vi "Init(Config) String Control Sink.vi"(7 "Str Refnum":refnum<vi>, 8 "error in (no error)":errorcluster, 9 "iName":string, 10 "iType":string) -> (0 "error out":errorcluster, 3 "String Control Sink out":refnum<class "String Control Sink.lvclass">)   [LabVIEW 2016, in "Stream Log.lvlib" / "String Control Sink.lvclass"]
doc: "--\nCopyright © 2017 Composed SystemsI All rights reserved.\n\nAuthor: Jon McBee <jon.mcbee@composed.io>\n\nThis library is provided \"AS IS\" ,WITHOUT WARRANTIES OR\nCONDITIONS OF ANY KIND, either express or implied.\n\nComposed Systems -- composed.io\n\nStream 0.0.1.1\nJon McBee - Composed Systems\nCopyright (c) 2017, Composed Systems"
uses:
  <userlib>/Composed Systems/Stream/Log/String Control Sink/String Control Sink.lvclass
  C:/Program Files (x86)/National Instruments/LabVIEW 2016/user.lib/Composed Systems/Stream/Actor/Actor Class/Ancestral Actor.lvclass
  <userlib>/Composed Systems/Stream/Actor/Actor Class/Ancestral Actor.lvclass/Ancestral Actor.ctl
  <userlib>/Composed Systems/Stream/Log/String Control Sink/String Control Sink.lvclass/String Control Sink.ctl
  <userlib>/Composed Systems/Stream/Actor/Actor Class/Ancestral Actor.lvclass
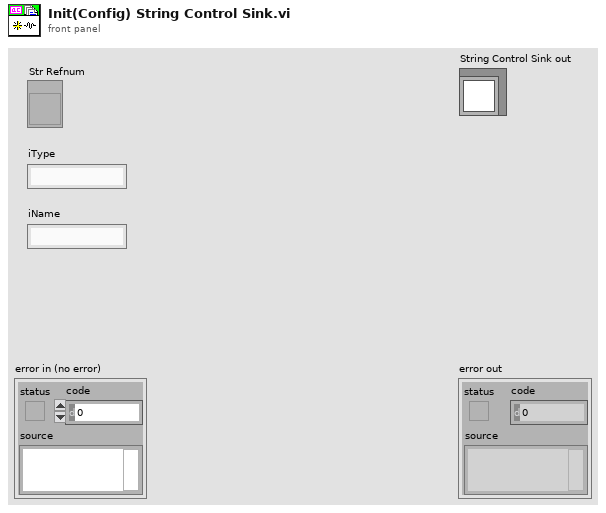
[diagram p1: front panel]
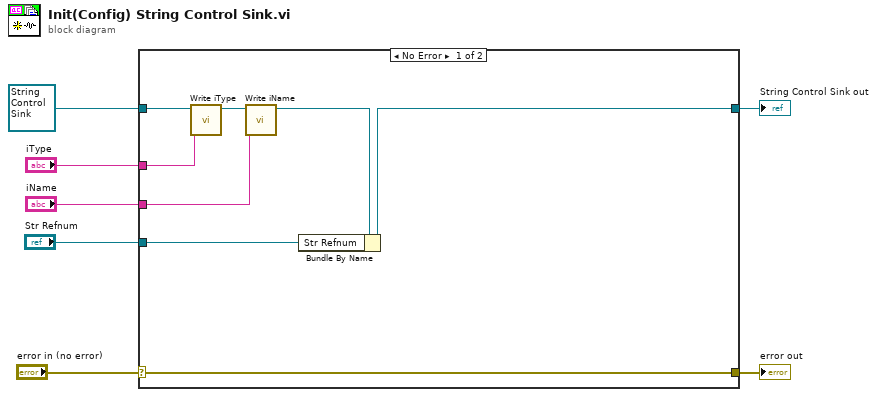
[diagram p0: block diagram]
diagram:
  n1 = case shown="No Error" "error in (no error)" {
    selector: "error in (no error)" -> [w15 w17]
    tunnel: [w15 w17] -> w6
    tunnel: [w9 w16] -> w4
    tunnel: refnum<class "String Control Sink.lvclass"> refnum ("String Control Sink in") -> [w13 w16]
    tunnel: "iType" -> [w12 _]
    tunnel: "iName" -> [w11 _]
    tunnel: "Str Refnum" -> [w8 _]
    frame No Error {
      n2 = call <userlib>:"Write iType.vi"("iType"=w12, "Ancestral Actor in"=w13) -> ("Ancestral Actor out"=w14:refnum<class "String Control Sink.lvclass">)  [unwired: 8 in, 1 out]
      n3 = call <userlib>:"Write iName.vi"("iName"=w11, "Ancestral Actor in"=w14) -> ("Ancestral Actor out"=w10:refnum<class "String Control Sink.lvclass">)  [unwired: 8 in, 1 out]
      n4 = Bundle By Name(cluster=w10, "Str Refnum"=w8) -> (w9:refnum<class "String Control Sink.lvclass">)
    }
    frame Error {
    }
  }
  "error out" <- w6
  "String Control Sink out" <- w4
